vi "Parse JSON and Add.vi"(8 "Error In":errorcluster, 10 "JSON String In":string="{\n    \"first\": \"2.5\",\n     \"second\": \"3.5\"\n}") -> (0 "Error Out":errorcluster, 2 "JSON String Out":string)   [LabVIEW 2014, in "lvwd-components-start-calc.lvlib"]
doc: "This VI parses the data that was POSTed to the /lvwd-components-start/calc/add endpoint. We expect the data format to be JSON so it is parsed as JSON, added together and returned as JSON. \n\n<B>Awesomeness:</B> Notice how we have seperated the Web Services specific VIs (Get Post Data, Write Response, etc) from the logic contained by this VI. This makes testing much easier. For example, press run on this VI to see it parse the JSON that was set as the default value and see the generated response that would be sent back to the client."
uses:
  lvwd-components-start-calc.lvlib
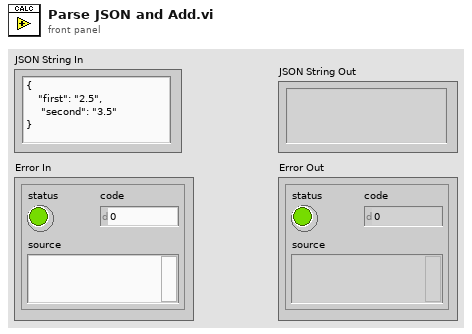
[diagram p1: front panel]
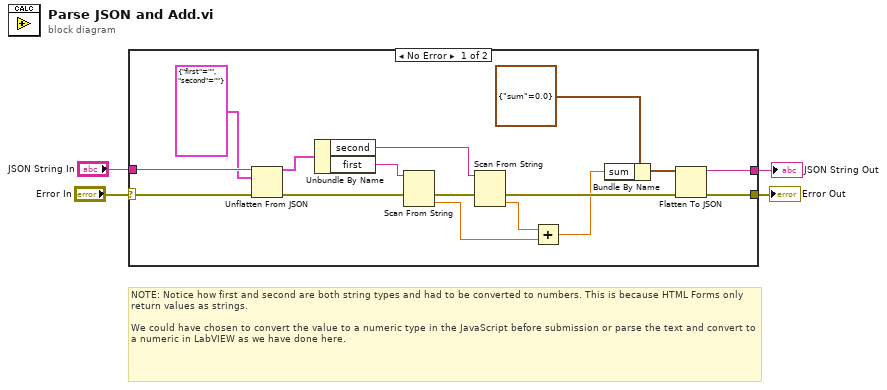
[diagram p0: block diagram]
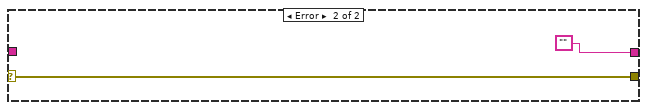
[diagram p2: hidden frame]
diagram:
  # "NOTE: Notice how first and second are both string types and had to be converted to numbers. This is because HTML Forms only return values as strings.\n\nWe could have chosen to convert the value to a numeric type in the JavaScript before submission or parse the text and convert to a numeric in LabVIEW as we have done here."
  n1 = case shown="No Error" "Error In" {
    selector: "Error In" -> [w17 w22]
    tunnel: "JSON String In" -> [w20 _]
    tunnel: [w9 w22] -> w2
    tunnel: [w5 ""] -> w1
    frame No Error {
      n2 = Unflatten From JSON(JSON string=w20, type and defaults=cluster{"first":string, "second":string} {"first"="", "second"=""}, error in (no error)=w17) -> (value=w18:cluster{"first":string, "second":string}, error out=w16:errorcluster)  [unwired: 4 in]
      n3 = Unbundle By Name(w18) -> ("second"=w11:string, "first"=w15:string)
      n4 = Scan From String(input string=w15, error in=w16) -> (error out=w14:errorcluster, output 1=w12:dbl)  [unwired: 3 in, 2 out]
      n5 = Scan From String(input string=w11, error in=w14) -> (error out=w10:errorcluster, output 1=w13:dbl)  [unwired: 3 in, 2 out]
      n6 = Add(x=w13, y=w12) -> (x+y=w6:dbl)
      n7 = Bundle By Name(cluster=cluster{"sum":dbl} {"sum"=0.0}, "sum"=w6) -> (w8:cluster{"sum":dbl})
      n8 = Flatten To JSON(anything=w8, error in (no error)=w10) -> (JSON string=w5:string, 11:w9:errorcluster)  [unwired: 1 in]
    }
    frame Error {
    }
  }
  "Error Out" <- w2
  "JSON String Out" <- w1
